vi "二维行数转换特定行号.vi"(1 "行数":i32) -> (0 "目标温度行号":i32)   [LabVIEW 2015]
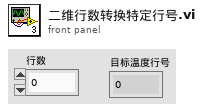
[diagram p1: front panel]
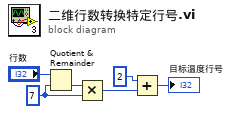
[diagram p0: block diagram]
diagram:
  w2 = 7
  n1 = Quotient & Remainder(x="行数", y=w2) -> (floor(x/y)=w1:i32)  [unwired: 1 out]
  n2 = Multiply(x=w1, y=w2) -> (x*y=w4:i32)
  n3 = Add(x=2, y=w4) -> (x+y=→"目标温度行号":i32)
